vi "midiMessageConstant--ContinuousController.vi"() -> (2 "Message":u8 format="%.0x")   [LabVIEW 2020, in "midi.lvclass"]
uses:
  midi.lvclass
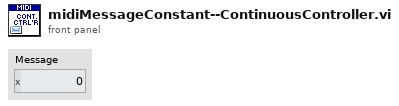
[diagram p1: front panel]
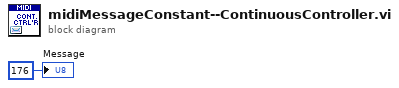
[diagram p0: block diagram]
diagram:
  "Message" <- u8 176 ("Message")
